vi "Laser349_RS232_End.vi"(8 "error in (no error)":errorcluster, 11 "Laser349 in":refnum<class "Laser349.lvclass">) -> (0 "error out":errorcluster, 3 "Laser349 out":refnum<class "Laser349.lvclass">)   [LabVIEW 2018, in "Laser349.lvclass"]
uses:
  Laser349.lvclass
  Laser349.lvclass/Laser349.ctl
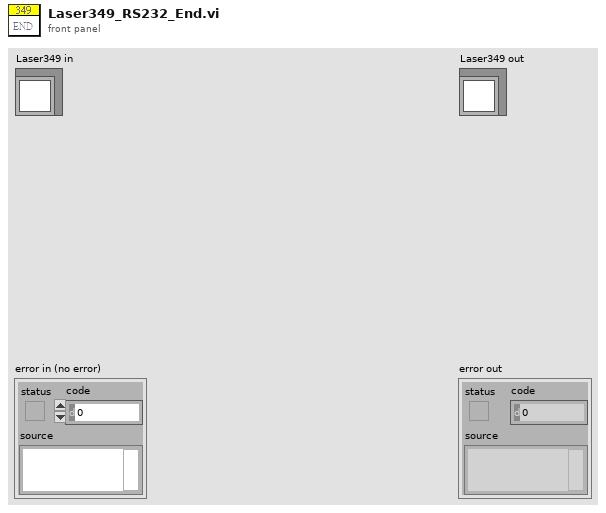
[diagram p1: front panel]
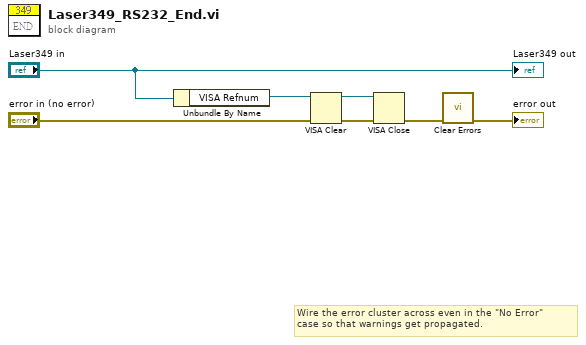
[diagram p0: block diagram]
diagram:
  # "Wire the error cluster across even in the \"No Error\"\ncase so that warnings get propagated."
  n1 = Unbundle By Name("Laser349 in") -> ("VISA Refnum"=w7:refnum<visa-resource-name>)
  n2 = VISA Clear(VISA resource name=w7, error in (no error)="error in (no error)") -> (VISA resource name out=w6:refnum<visa-resource-name>, error out=w5:errorcluster)
  n3 = VISA Close(VISA resource name=w6, error in (no error)=w5) -> (error out=w2:errorcluster)
  n4 = call <vilib>:"Clear Errors.vi"("error in (no error)"=w2) -> ("error out"=→"error out":errorcluster)  [unwired: 5 in, 1 out]
  "Laser349 out" <- "Laser349 in"
